vi "main.vi"(8 "error in (no error)":errorcluster) -> (0 "error out":errorcluster)   [LabVIEW 2015, in "lv-interface-dom-nre.lvlib"]
uses:
  lv-interface-dom-nre.lvlib
  lv-interface-sub-common/_controls/interface_selection.ctl
  public/_controls/fg_command.ctl
  lv-interface-sub-common/_controls/fg_command.ctl
  private/_controls/hmi_references.ctl
  private/_controls/hmi_states.ctl
  private/_controls/event_common.ctl
  private/_controls/event_common_command.ctl
  private/_controls/event_interface.ctl
  private/_controls/event_interface_command.ctl
  private/_controls/menu_selection.ctl
  lv-interface-sub-common/lv-interface-sub-common.lvlib
panel:
  out "time":dbl format="%<%H:%M:%S\n%m/%d/%y>T"
  out "random_number":dbl
  in  "switch_unload":bool
  in  "interface":T1=enum."sub_interface_1"
  in  "focus_unfocus":bool
  # "test"
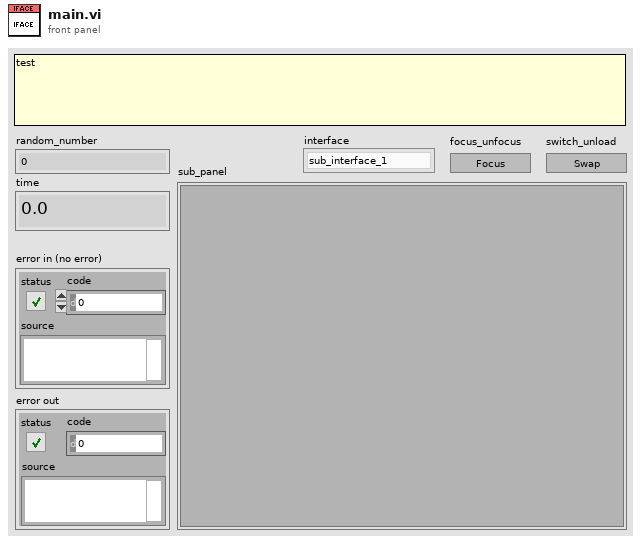
[diagram p1: front panel]
types:
  T1 = typedef "lv-interface-sub-common.lvlib/interface_selection.ctl" = enum16{"<interface>", "sub_interface_1", "sub_interface_2", "<null>"}
  T2 = typedef "lv-interface-sub-common.lvlib/fg_command.ctl" = enum16{"<fg_command>", "initialize", "read", "write", "shutdown", "<null>"}
  T3 = typedef "lv-interface-dom-nre.lvlib/fg_command.ctl" = enum16{"<fg_command>", "initialize", "read", "write", "shutdown", "<null>"}
  T4 = typedef "lv-interface-dom-nre.lvlib/hmi_references.ctl" = cluster{"vi_reference":refnum<vi>, "sub_panel":refnum<vi>}
  T5 = typedef "lv-interface-dom-nre.lvlib/event_interface.ctl" = cluster{"command":T6, "data":variant}
  T6 = typedef "lv-interface-dom-nre.lvlib/event_interface_command.ctl" = enum16{"<event_interface_cmd>", "defer_panel_updates", "undefer_panel_updates", "load_interface", "<null>"}
  T7 = typedef "lv-interface-dom-nre.lvlib/event_common.ctl" = cluster{"command":T8, "data":variant}
  T8 = typedef "lv-interface-dom-nre.lvlib/event_common_command.ctl" = enum16{"<event_common_cmd>", "die", "<null>"}
  T9 = typedef "lv-interface-dom-nre.lvlib/hmi_states.ctl" = enum16{"<hmi_states>", "initialize", "checkui", "updateui", "shutdown", "<null>"}
  T10 = typedef "lv-interface-dom-nre.lvlib/menu_selection.ctl" = enum16{"<menu>", "file_exit", "help_about", "<null>"}
  T11 = typedef "lv-interface-dom-nre.lvlib/interface_refnum.ctl" = refnum<vi>
  T12 = typedef "interface_dom_nre.lvlib/interface_selection.ctl" = enum16{"<interface>", "sub_interface_1", "sub_interface_2", "<null>"}
  T13 = typedef "interface_dom_nre.lvlib/event_to_dom_command.ctl" = enum16{"<to_dom_cmd>", "load_interface", "die", "<null>"}
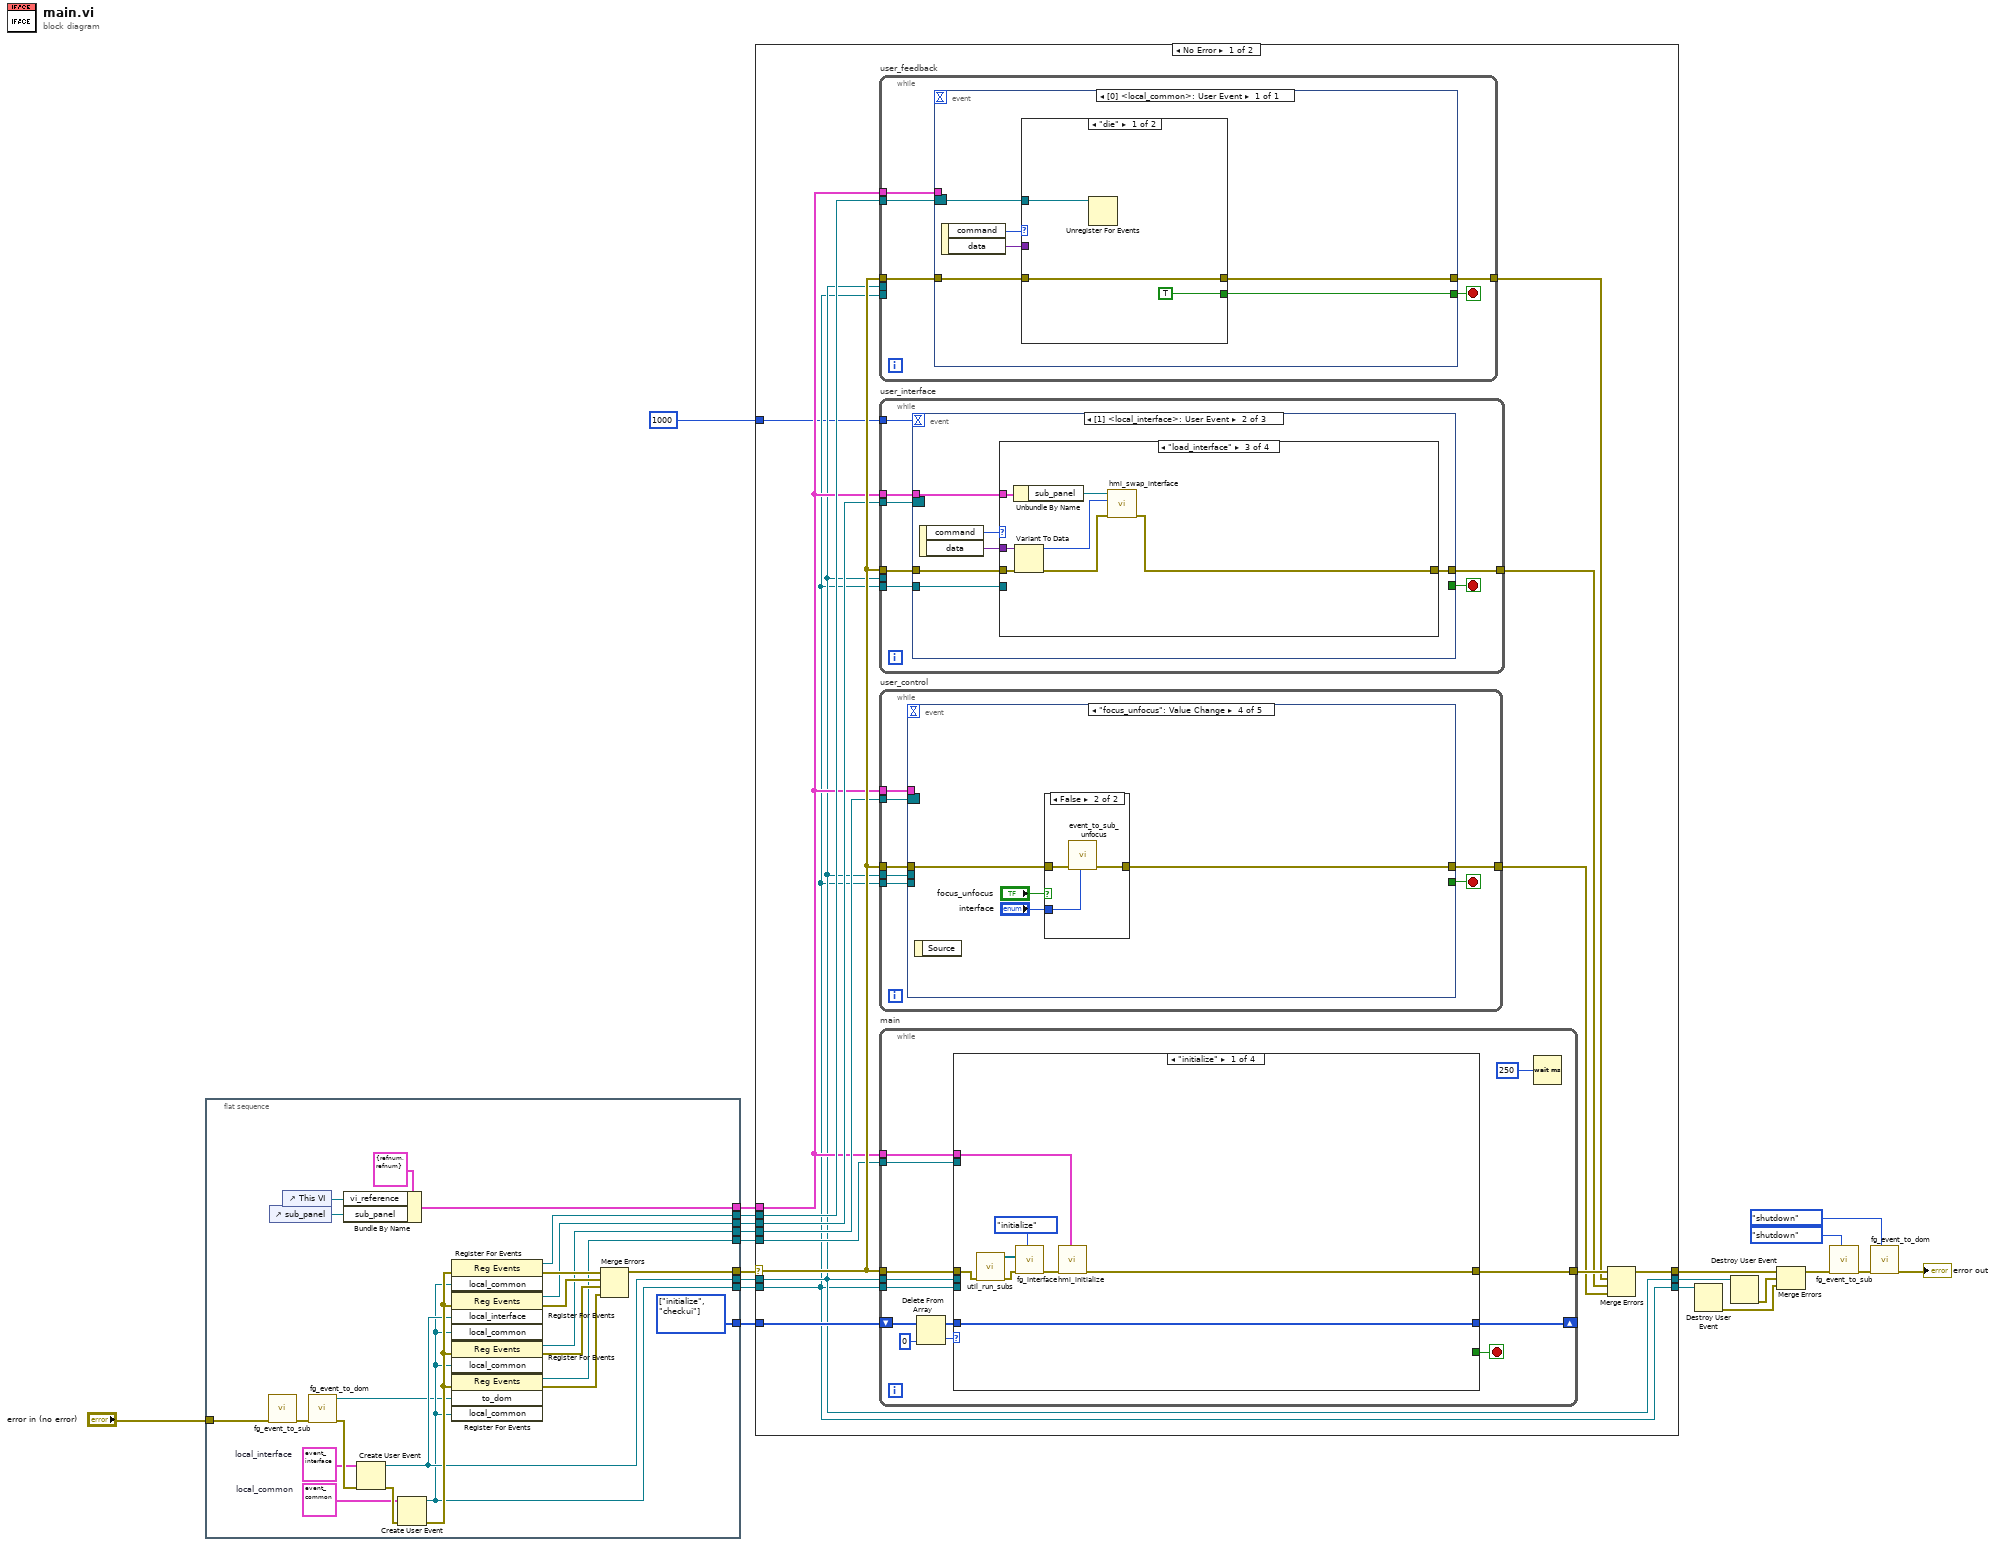
[diagram p0: block diagram]
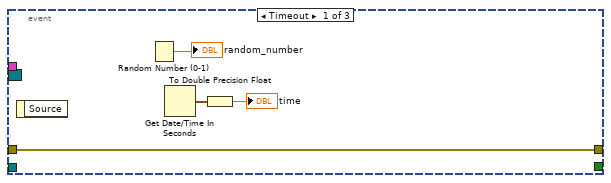
[diagram p3: hidden frame]
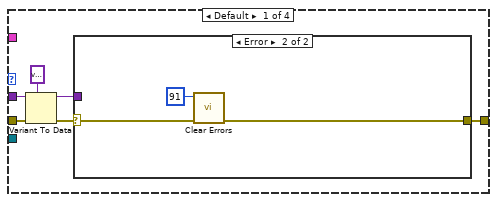
[diagram p4: hidden frame]
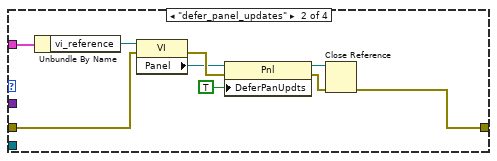
[diagram p6: hidden frame]
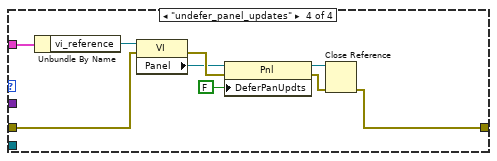
[diagram p7: hidden frame]
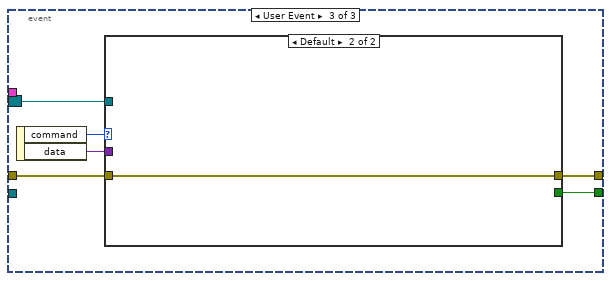
[diagram p8: hidden frame]
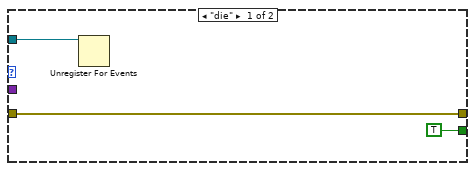
[diagram p9: hidden frame]
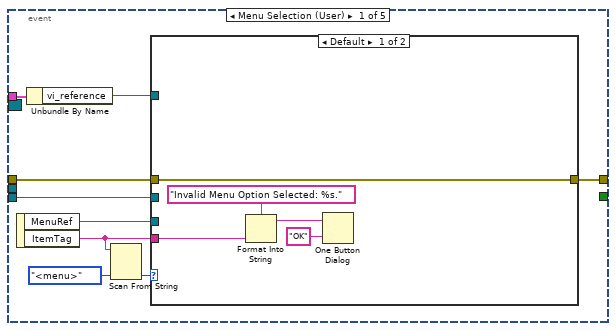
[diagram p10: hidden frame]
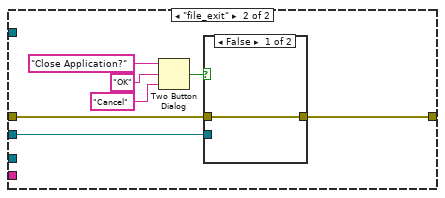
[diagram p11: hidden frame]
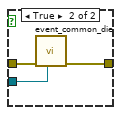
[diagram p12: hidden frame]
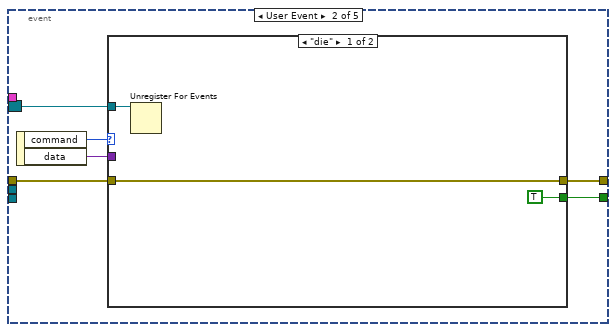
[diagram p13: hidden frame]
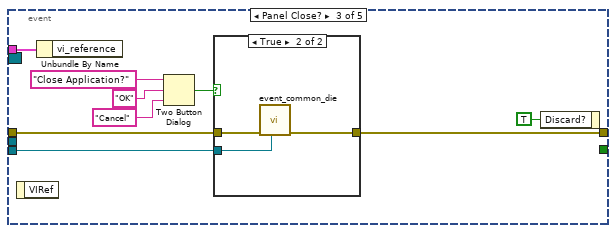
[diagram p15: hidden frame]
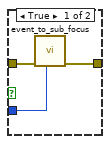
[diagram p17: hidden frame]
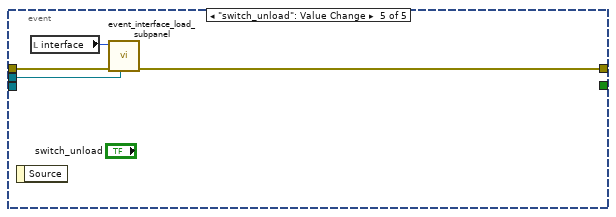
[diagram p18: hidden frame]
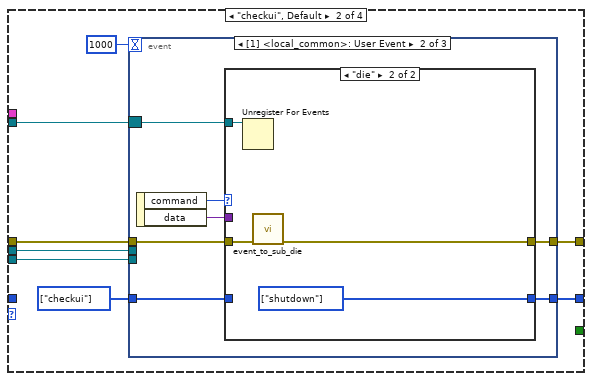
[diagram p19: hidden frame]
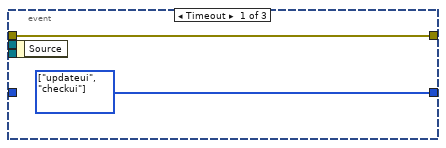
[diagram p20: hidden frame]
diagram:
  n1 = flat-sequence {
    tunnel: [w36] -> w21
    tunnel: [w35] -> w20
    tunnel: [w39] -> w19
    tunnel: "error in (no error)" -> [w24]
    tunnel: [w34] -> w17
    tunnel: [w33] -> w16
    tunnel: [w31] -> w15
    tunnel: [w25] -> w13
    tunnel: [w28] -> w14
    tunnel: [w27] -> w7
    frame #0 {
      w29 = T5 {"command"=enum."<event_interface_cmd>", "data"=variant}  # local_interface
      w30 = T7 {"command"=enum."<event_common_cmd>", "data"=variant}  # local_common
      w39 = T9[] [enum."initialize", enum."checkui"] items=["<hmi_states>", "initialize", "checkui", "updateui", "shutdown", "<null>"]
      n2 = call "fg_event_to_sub.vi"("error in (no error)"=w24) -> ("error out"=w23:errorcluster)  [unwired: 8 in, 2 out]
      n3 = control-ref of="sub_panel"() -> (w26:refnum<vi>)
      n4 = control-ref of="This VI"() -> (w32:refnum<vi>)
      n5 = call "fg_event_to_dom.vi"("error in (no error)"=w23) -> ("error out"=w45:errorcluster, "to_dom"=w22:refnum<user-event>)  [unwired: 8 in, 1 out]
      n6 = Bundle By Name(cluster=T4 {"vi_reference"=refnum, "sub_panel"=refnum}, "vi_reference"=w32, "sub_panel"=w26) -> (w31:T4)
      n7 = Create User Event(user event datatype=w29, error in=w45) -> (user event=w28:refnum<user-event>, error out=w43:errorcluster)
      n8 = Create User Event(user event datatype=w30, error in=w43) -> (user event=w25:refnum<user-event>, error out=w42:errorcluster)
      n9 = register-events(error in=w42, w25) -> (reference out=w27:refnum<event-registration>, error out=w44:errorcluster)  [unwired: 1 in]
      n10 = register-events(error in=w42, w28, w25) -> (reference out=w33:refnum<event-registration>, error out=w41:errorcluster)  [unwired: 1 in]
      n11 = register-events(error in=w42, w25) -> (reference out=w35:refnum<event-registration>, error out=w38:errorcluster)  [unwired: 1 in]
      n12 = register-events(error in=w42, w22, w25) -> (reference out=w34:refnum<event-registration>, error out=w37:errorcluster)  [unwired: 1 in]
      n13 = Merge Errors(w44, w41, w38, w37) -> (w36:errorcluster)
    }
  }
  n14 = case shown="No Error" w21 {
    selector: w21 -> [w60 w289]
    tunnel: w20 -> [w53 w285]
    tunnel: w19 -> [w55 _]
    tunnel: [w51 w289] -> w10
    tunnel: w17 -> [w54 w284]
    tunnel: w16 -> [w52 w286]
    tunnel: w15 -> [w50 _]
    tunnel: w14 -> [w49 w288]
    tunnel: w13 -> [w48 w287]
    tunnel: [w49 w288] -> w11
    tunnel: [w48 w287] -> w12
    tunnel: w7 -> [w59 w283]
    tunnel: 1000 -> [w46 _]
    frame No Error {
      n15 = while "user_feedback" {
        tunnel: [w65] -> w47
        tunnel: w60 -> [w64]
        tunnel: w59 -> [w63]
        tunnel: w50 -> [w62]
        tunnel: w49 -> [_]
        tunnel: w48 -> [_]
        stop <- w61 stop-if-true
        n16 = event shown="[0] <local_common>: User Event" {
          selector: w63 -> [w71]
          dyn-events: _ -> [_]
          timeout: _ -> [_]
          tunnel: [w68] -> w65
          tunnel: w64 -> [w69]
          tunnel: w62 -> [_]
          tunnel: [w67] -> w61
          event User Event {
            n17 = event-data() -> ("command"=w70:T8, "data"=w66:variant)  [unwired: 1 in]
            n18 = case shown="\"die\"" w70 {
              tunnel: w69 -> [w73 w75]
              tunnel: [w73 w75] -> w68
              tunnel: [TRUE _] -> w67
              tunnel: w71 -> [w72 _]
              tunnel: w66 -> [_ _]
              frame "die" {
                n19 = Unregister For Events(event registration refnum=w72) -> ()  [unwired: 1 in, 1 out]
              }
              frame Default {
              }
            }
          }
        }
      }
      n20 = while "user_interface" {
        tunnel: w60 -> [w82]
        tunnel: [w80] -> w56
        tunnel: w52 -> [w79]
        tunnel: w49 -> [_]
        tunnel: w48 -> [w78]
        tunnel: w50 -> [w77]
        tunnel: w46 -> [w76]
        stop <- w81 stop-if-true
        n21 = event shown="[1] <local_interface>: User Event" {
          selector: w79 -> [_ _ w129]
          dyn-events: _ -> [_ _ _]
          timeout: w76 -> [_ _ _]
          tunnel: w82 -> [w86 w90 w132]
          tunnel: [w86 w89 w131] -> w80
          tunnel: [_ _ w130] -> w81
          tunnel: w78 -> [_ w88 _]
          tunnel: w77 -> [_ w87 _]
          event Timeout {
            n22 = event-data() -> ()  [unwired: 1 in, 1 out]
            n23 = Random Number (0-1)() -> (number: 0 to 1=→"random_number":dbl)
            n24 = Get Date/Time In Seconds() -> (seconds since 1Jan1904=w83:timestamp)
            n25 = To Double Precision Float(number=w83) -> (double precision float=→"time":dbl)
          }
          event User Event {
            n26 = event-data() -> ("command"=w92:T6, "data"=w91:variant)  [unwired: 1 in]
            n27 = case shown="\"load_interface\"" w92 {
              tunnel: w90 -> [w97 w106 w117 w122]
              tunnel: [w93 w105 w115 w119] -> w89
              tunnel: w91 -> [w98 _ w118 _]
              tunnel: w88 -> [_ _ _ _]
              tunnel: w87 -> [_ w104 w113 w121]
              frame Default {
                n28 = Variant To Data(error in=w97, type=variant, Variant=w98) -> (data=w94:variant, error out=w96:errorcluster)
                n29 = case shown="Error" w96 {
                  selector: w96 -> [w99 w102]
                  tunnel: w94 -> [_ _]
                  tunnel: [w99 w101] -> w93
                  frame No Error {
                  }
                  frame Error {
                    n30 = call <vilib>:"Clear Errors.vi"("error in (no error)"=w102, "specific error code to clear (0: all)"=91) -> ("error out"=w101:errorcluster)  [unwired: 4 in, 1 out]
                  }
                }
              }
              frame "defer_panel_updates" {
                n31 = Unbundle By Name(w104) -> ("vi_reference"=w103:refnum<vi>)
                n32 = property class="VI"(reference=w103, error in=w106) -> (error out=w111:errorcluster, "Panel"=w107:refnum<vi>)  [unwired: 1 out]
                n33 = property class="Pnl"(reference=w107, error in=w111, "DeferPanUpdts"=TRUE ("Defer Panel Updates")) -> (reference out=w109:refnum<vi>, error out=w108:errorcluster)
                n34 = Close Reference(reference=w109, error in (no error)=w108) -> (error out=w105:errorcluster)
              }
              frame "load_interface" {
                n35 = Unbundle By Name(w113) -> ("sub_panel"=w112:refnum<vi>)
                n36 = Variant To Data(error in=w117, Variant=w118) -> (data=w114:T1, error out=w116:errorcluster)  [unwired: 1 in]
                n37 = call "hmi_swap_interface.vi"("error in (no error)"=w116, "interface"=w114, "subpanel_reference"=w112) -> ("error out"=w115:errorcluster)  [unwired: 8 in]
              }
              frame "undefer_panel_updates" {
                n38 = Unbundle By Name(w121) -> ("vi_reference"=w120:refnum<vi>)
                n39 = property class="VI"(reference=w120, error in=w122) -> (error out=w127:errorcluster, "Panel"=w123:refnum<vi>)  [unwired: 1 out]
                n40 = property class="Pnl"(reference=w123, error in=w127, "DeferPanUpdts"=FALSE ("Defer Panel Updates")) -> (reference out=w125:refnum<vi>, error out=w124:errorcluster)
                n41 = Close Reference(reference=w125, error in (no error)=w124) -> (error out=w119:errorcluster)
              }
            }
          }
          event User Event {
            n42 = event-data() -> ("command"=w133:T8, "data"=w128:variant)  [unwired: 1 in]
            n43 = case shown="Default" w133 {
              tunnel: w132 -> [w135 w137]
              tunnel: [w135 w137] -> w131
              tunnel: [TRUE _] -> w130
              tunnel: w129 -> [w134 _]
              tunnel: w128 -> [_ _]
              frame "die" {
                n44 = Unregister For Events(event registration refnum=w134) -> ()  [unwired: 1 in, 1 out]
              }
              frame Default {
              }
            }
          }
        }
      }
      n45 = while "user_control" {
        tunnel: w60 -> [w144]
        tunnel: [w142] -> w57
        tunnel: w53 -> [w141]
        tunnel: w49 -> [w139]
        tunnel: w48 -> [w138]
        tunnel: w50 -> [w140]
        stop <- w143 stop-if-true
        n46 = event shown="[3] \"focus_unfocus\": Value Change" {
          selector: w141 -> [_ w170 _ _ _]
          dyn-events: _ -> [_ _ _ _ _]
          timeout: _ -> [_ _ _ _ _]
          tunnel: w144 -> [w150 w174 w180 w196 w206]
          tunnel: [w148 w173 w187 w195 w203] -> w142
          tunnel: [_ w172 _ _ _] -> w143
          tunnel: w140 -> [w147 _ w186 _ _]
          tunnel: w139 -> [_ _ _ _ w204]
          tunnel: w138 -> [w145 _ w185 _ _]
          event Menu Selection (User) {
            n47 = event-data() -> ("MenuRef"=w151:refnum<k9>, "ItemTag"=w149:string)  [unwired: 1 in]
            n48 = Unbundle By Name(w147) -> ("vi_reference"=w146:refnum<vi>)
            n49 = Scan From String(input string=w149, default 1=menu_selection."<menu>" ("menu_selection")) -> (output 1=w152:T10)  [unwired: 3 in, 3 out]
            n50 = case shown="Default" w152 {
              tunnel: w151 -> [_ _]
              tunnel: w150 -> [w154 w159]
              tunnel: w149 -> [w158 _]
              tunnel: [w154 w165] -> w148
              tunnel: w146 -> [_ _]
              tunnel: w145 -> [_ w164]
              frame Default {
                n51 = Format Into String(format string="Invalid Menu Option Selected: %s.", w158) -> (resulting string=w156:string)  [unwired: 2 in, 1 out]
                n52 = One Button Dialog(message=w156, button name ("OK")="OK" ("boolean_text_1")) -> ()  [unwired: 1 out]
              }
              frame "file_exit" {
                n53 = Two Button Dialog(message="Close Application?" ("dialog_text"), 1:"Cancel" ("boolean_text_1"), 2:"OK" ("boolean_text_1")) -> (T button?=w160:bool)
                n54 = case shown="False" w160 {
                  tunnel: w159 -> [w166 w169]
                  tunnel: [w166 w168] -> w165
                  tunnel: w164 -> [_ w167]
                  frame False {
                  }
                  frame True {
                    n55 = call "event_common_die.vi"("local_common"=w167, "error in (no error)"=w169) -> ("error out"=w168:errorcluster)  [unwired: 9 in]
                  }
                }
              }
            }
          }
          event User Event {
            n56 = event-data() -> ("command"=w175:T8, "data"=w171:variant)  [unwired: 1 in]
            n57 = case shown="\"die\"" w175 {
              tunnel: w174 -> [w176 w179]
              tunnel: [w176 w179] -> w173
              tunnel: [TRUE _] -> w172
              tunnel: w171 -> [_ _]
              tunnel: w170 -> [w177 _]
              frame "die" {
                n58 = Unregister For Events(event registration refnum=w177) -> ()  [unwired: 1 in, 1 out]
              }
              frame Default {
              }
            }
          }
          event Panel Close? {
            n59 = event-data() -> ()  [unwired: 1 in, 1 out]
            n60 = Unbundle By Name(w186) -> ()  [unwired: 1 out]
            n61 = Two Button Dialog(message="Close Application?" ("dialog_text"), 1:"Cancel" ("boolean_text_1"), 2:"OK" ("boolean_text_1")) -> (T button?=w181:bool)
            n62 = case shown="True" w181 {
              tunnel: w180 -> [w189 w192]
              tunnel: [w189 w191] -> w187
              tunnel: w185 -> [_ w190]
              frame False {
              }
              frame True {
                n63 = call "event_common_die.vi"("local_common"=w190, "error in (no error)"=w192) -> ("error out"=w191:errorcluster)  [unwired: 9 in]
              }
            }
            n64 = event-data("Discard?"=TRUE) -> ()  [unwired: 1 in, 1 out]
          }
          event "focus_unfocus": Value Change {
            n65 = event-data() -> ()  [unwired: 1 in, 1 out]
            n66 = case shown="False" "focus_unfocus" {
              tunnel: w196 -> [w199 w202]
              tunnel: [w198 w201] -> w195
              tunnel: "interface" -> [w197 w200]
              frame True {
                n67 = call "event_to_sub_focus.vi"("interface"=w197, "error in (no error)"=w199) -> ("error out"=w198:errorcluster)  [unwired: 9 in]
              }
              frame False {
                n68 = call "event_to_sub_unfocus.vi"("interface"=w200, "error in (no error)"=w202) -> ("error out"=w201:errorcluster)  [unwired: 9 in]
              }
            }
          }
          event "switch_unload": Value Change {
            n69 = event-data() -> ()  [unwired: 1 in, 1 out]
            n70 = local read "interface"() -> (w205:T1)
            n71 = call "event_interface_load_subpanel.vi"("event_interface"=w204, "error in (no error)"=w206, "interface"=w205) -> ("error out"=w203:errorcluster)  [unwired: 8 in]
          }
        }
      }
      n72 = while "main" {
        shift-right: [w211] -> _
        shift-left: w55 -> [w218]
        tunnel: w54 -> [w212]
        tunnel: w60 -> [w214]
        tunnel: [w210] -> w58
        tunnel: w50 -> [w209]
        tunnel: w48 -> [w208]
        tunnel: w49 -> [w207]
        stop <- w213 stop-if-true
        n73 = Delete From Array(array=w218, index=0) -> (deleted portion=w216:T9, array with subset deleted=w215:T9[])  [unwired: 1 in]
        n74 = case shown="\"initialize\"" w216 {
          tunnel: w215 -> [w227 _ w274 _]
          tunnel: w214 -> [w222 w234 w273 w281]
          tunnel: [_ _ _ TRUE] -> w213
          tunnel: [w225 w233 w273 w275] -> w210
          tunnel: [w227 w232 w274 w280] -> w211
          tunnel: w212 -> [_ w230 _ _]
          tunnel: w209 -> [w226 _ _ w279]
          tunnel: w208 -> [_ w228 _ _]
          tunnel: w207 -> [_ w229 _ _]
          frame "initialize" {
            n75 = call "util_run_subs.vi"("error in (no error)"=w222) -> ("error out"=w221:errorcluster, "interface []"=w223:T11[])  [unwired: 9 in]
            n76 = call "fg_interface.vi"("fg_command"=fg_command."initialize", "error in (no error)"=w221, "interface [] in"=w223) -> ("error out"=w220:errorcluster)  [unwired: 6 in, 2 out]
            n77 = call "hmi_initialize.vi"("hmi_references"=w226, "error in (no error)"=w220) -> ("error out"=w225:errorcluster)  [unwired: 9 in]
          }
          frame "checkui", Default {
            w231 = T9[] [enum."checkui"] items=["<hmi_states>", "initialize", "checkui", "updateui", "shutdown", "<null>"]
            n78 = event shown="[1] <local_common>: User Event" {
              selector: w230 -> [_ w238 _]
              dyn-events: _ -> [_ _ _]
              timeout: 1000 -> [_ _ _]
              tunnel: w234 -> [w237 w242 w257]
              tunnel: [w237 w239 w254] -> w233
              tunnel: [w236 w240 w255] -> w232
              tunnel: w231 -> [_ w241 w256]
              tunnel: w229 -> [_ _ w252]
              tunnel: w228 -> [_ _ w251]
              event Timeout {
                w236 = T9[] [enum."updateui", enum."checkui"] items=["<hmi_states>", "initialize", "checkui", "updateui", "shutdown", "<null>"]
                n79 = event-data() -> ()  [unwired: 1 in, 1 out]
              }
              event User Event {
                n80 = event-data() -> ("command"=w244:T8, "data"=w243:variant)  [unwired: 1 in]
                n81 = case shown="\"die\"" w244 {
                  tunnel: [w246 w250] -> w240
                  tunnel: w241 -> [w246 _]
                  tunnel: w242 -> [w245 w248]
                  tunnel: [w245 w247] -> w239
                  tunnel: w243 -> [_ _]
                  tunnel: w238 -> [_ w249]
                  frame Default {
                  }
                  frame "die" {
                    w250 = T9[] [enum."shutdown"] items=["<hmi_states>", "initialize", "checkui", "updateui", "shutdown", "<null>"]
                    n82 = Unregister For Events(event registration refnum=w249) -> ()  [unwired: 1 in, 1 out]
                    n83 = call "event_to_sub_die.vi"("error in (no error)"=w248) -> ("error out"=w247:errorcluster)  [unwired: 10 in]
                  }
                }
              }
              event User Event {
                n84 = event-data() -> ("interface"=w253:T12, "command"=w259:T13, "data"=w258:variant)  [unwired: 1 in]
                n85 = case shown="\"die\"" w259 {
                  tunnel: [w261 w268 w272] -> w255
                  tunnel: w256 -> [w261 w268 w272]
                  tunnel: w257 -> [w260 w266 w270]
                  tunnel: [w260 w262 w269] -> w254
                  tunnel: w258 -> [_ w267 _]
                  tunnel: w253 -> [_ _ _]
                  tunnel: w252 -> [_ w263 _]
                  tunnel: w251 -> [_ _ w271]
                  frame Default {
                  }
                  frame "load_interface" {
                    n86 = Variant To Data(error in=w266, Variant=w267) -> (data=w265:T1, error out=w264:errorcluster)  [unwired: 1 in]
                    n87 = call "event_interface_load_subpanel.vi"("event_interface"=w263, "error in (no error)"=w264, "interface"=w265) -> ("error out"=w262:errorcluster)  [unwired: 8 in]
                  }
                  frame "die" {
                    n88 = call "event_common_die.vi"("local_common"=w271, "error in (no error)"=w270) -> ("error out"=w269:errorcluster)  [unwired: 9 in]
                  }
                }
              }
            }
          }
          frame "updateui" {
          }
          frame "shutdown" {
            w280 = T9[] [enum."shutdown"] items=["<hmi_states>", "initialize", "checkui", "updateui", "shutdown", "<null>"]
            n89 = call "hmi_shutdown.vi"("hmi_references"=w279, "error in (no error)"=w281) -> ("error out"=w278:errorcluster)  [unwired: 9 in]
            n90 = call "fg_interface.vi"("error in (no error)"=w278) -> ("error out"=w277:errorcluster, "interface [] out"=w276:T11[])  [unwired: 8 in, 1 out]
            n91 = call "util_stop_subs.vi"("error in (no error)"=w277, "interface []"=w276) -> ("error out"=w275:errorcluster)  [unwired: 9 in]
          }
        }
        n92 = Wait (ms)(milliseconds to wait=u32 250) -> ()  [unwired: 1 out]
      }
      n93 = Merge Errors(w58, w47, w56, w57) -> (w51:errorcluster)
    }
    frame Error {
      n94 = Unregister For Events(event registration refnum=w284) -> ()  [unwired: 1 in, 1 out]
      n95 = Unregister For Events(event registration refnum=w285) -> ()  [unwired: 1 in, 1 out]
      n96 = Unregister For Events(event registration refnum=w286) -> ()  [unwired: 1 in, 1 out]
      n97 = Unregister For Events(event registration refnum=w283) -> ()  [unwired: 1 in, 1 out]
    }
  }
  n98 = Destroy User Event(user event=w12) -> (error out=w8:errorcluster)  [unwired: 1 in]
  n99 = Destroy User Event(user event=w11) -> (error out=w9:errorcluster)  [unwired: 1 in]
  n100 = Merge Errors(w10, w9, w8) -> (w5:errorcluster)
  n101 = call "fg_event_to_sub.vi"("fg_command"=fg_command."shutdown", "error in (no error)"=w5) -> ("error out"=w6:errorcluster)  [unwired: 7 in, 2 out]
  n102 = call "fg_event_to_dom.vi"("fg_command"=fg_command."shutdown", "error in (no error)"=w6) -> ("error out"=→"error out":errorcluster)  [unwired: 7 in, 2 out]
